vi "P2P High-Speed Stream to Disk.vi"() -> ()   [LabVIEW 2023]
doc: "Shows best-practices for streaming high-speed data to disk from a 791x coprocessor module."
uses:
  <vilib>/userDefined/Silver/nirio_resource_slv.ctl
  SubVIs/UI_indicators.ctl
  <instrlib>/_niInstr/Streaming/v1/Common/Stream State.ctl
  <vilib>/userDefined/niP2PState.ctl
  <vilib>/FPGAPlugInAG/PXIe-7915/niLvFpga_Open_PXIe-7915.vi
  <vilib>/rvi/interface/common/dynamic/niFpgaDynamicAddResources.vi
  <vilib>/FPGAPlugInAG/Dynamic/niLvFpga_P2PGetEndpoint_Dynamic.vi
  <vilib>/Utility/error.llb/Error Cluster From Error Code.vi
  <vilib>/rvi/errors/niLvFpgaAdjustHostInterfaceError.vi
  <vilib>/FPGAPlugInAG/Dynamic/niLvFpga_Close_Dynamic.vi
  <vilib>/rvi/interface/nirviOpenFPGA/nirviOpenFPGA.xnode
  FPGA Bitfiles/PXIe-791X_Getting_Started.lvbitx
  <vilib>/rvi/interface/nirviMethod/nirviMethod.xnode
  <vilib>/rvi/interface/nirviReadWriteControl/nirviReadWriteControl.xnode
  <vilib>/rvi/interface/nirviCloseFPGA/nirviCloseFPGA.xnode
  <instrlib>/_niInstr/Streaming/v1/Host/niInstr Streaming v1 Host.lvlib
  <vilib>/rvi/errors/niLvFpgaMergeErrorWithErrorCode.vi
  <instrlib>/_niInstr/Streaming/v1/Common/niInstr Streaming v1 Common.lvlib
  <instrlib>/FlexRIO/API/Host/v1/NI FlexRIO API v1.lvlib
  <resource>/objmgr/niflexrioapi.rc
  <resource>/objmgr/PeerToPeerStream.rc
  NiFpgaLv.dll
  <vilib>/rvi/interface/Simulation/niFpgaSimulationCallBeginRW.vi
  <vilib>/FPGAPlugInAG/Dynamic/niLvFpga_AcquireReadRegionFifo_Dynamic.vi
  <vilib>/FPGAPlugInAG/Dynamic/niLvFpga_StopFifo_Dynamic.vi
panel:
  out "P2P State":T1
  in  "P2P Data Source":T2="RIO1"
  out "FPGA Temperature (degC)":dbl(slide) scale=0.0..95.0
  out "Total Power Consumed (W)":dbl(slide) scale=0.0..38.25
  out "Stream Status":T3
  in  "Max File Size (GB)":dbl=2.0 format="%#_g GB"
  out "Actual Host Buffer Depth (Samples)":u32=4194304 format="%.0f S"
  in  "File Write Block Size (Samples per Read)":u32=262144 format="%.0f S"
  in  "Host Buffer Depth (# of File Write Blocks)":u32=16 format="%.0f Blocks"
  in  "TDMS File Path":path=path "C:/temp.tdms"
  in  "Total Blocks to Record (# of File Write Blocks)":u64=256 format="%.0p"
  in  "791x Coprocessor FPGA":T2="RIO0"
  # "Configuration"
  # "Power & Temperature"
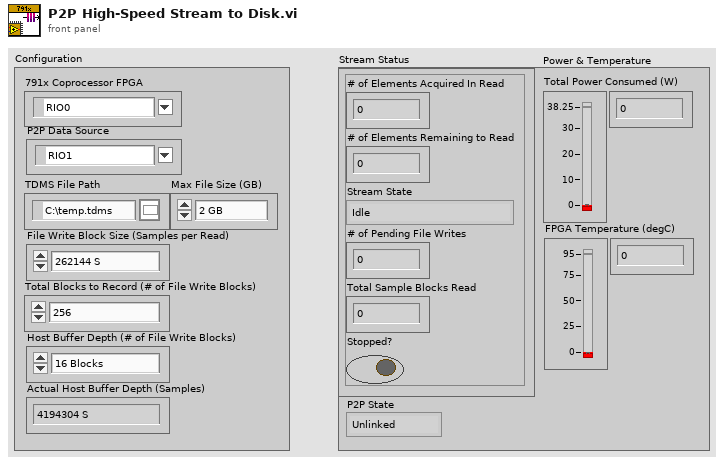
[diagram p1: front panel]
types:
  T1 = typedef "niP2PState.ctl" = enum32{"Unlinked", "Disabled", "Enabled", "Flushing"}
  T2 = typedef "nirio_resource_slv.ctl" = tag
  T3 = typedef "UI_indicators.ctl" = cluster{"# of Elements Acquired In Read":u32, "# of Elements Remaining to Read":u32, "Stream State":T4, "# of Pending File Writes":u32, "Total Sample Blocks Read":i32, "Stopped?":bool}
  T4 = typedef "niInstr Streaming v1 Common.lvlib/Stream State.ctl" = enum8{"Idle", "Finite Transfer", "Continuous", "Done", "Error", "Not Ready", "Cancel"}
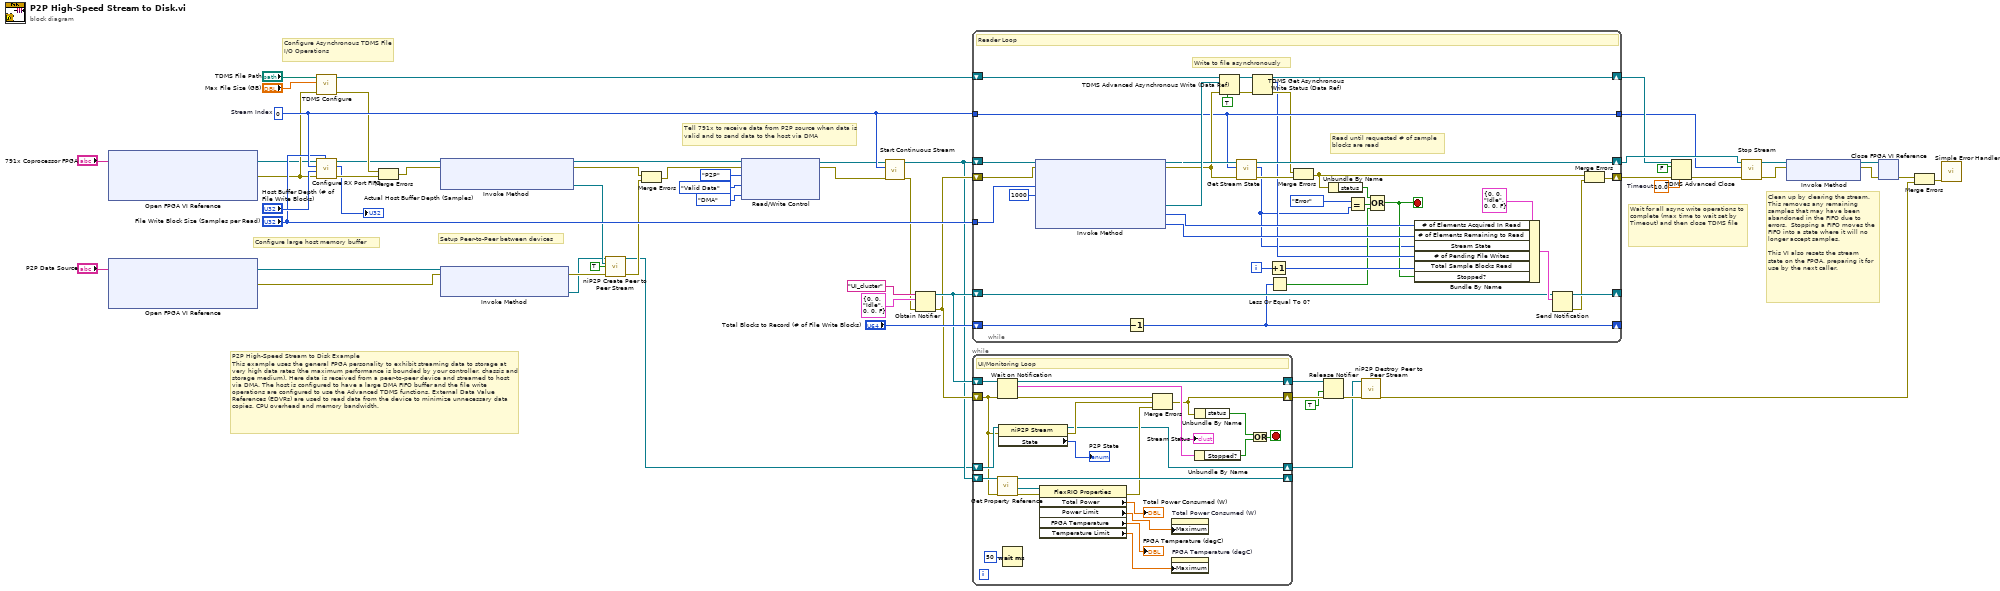
[diagram p0: block diagram]
diagram:
  w39 = 10.0  # Timeout
  w49 = 0  # Stream Index
  # "P2P High-Speed Stream to Disk Example\nThis example uses the general FPGA personality to exhibit streaming data to storage at very high data rates (the maximum performance is bounded by your controller, chassis and storage medium). Here data is received from a peer-to-peer device and streamed to host via DMA. The host is configured to have a large DMA FIFO buffer and the file write operations are configured to use the Advanced TDMS functions. External Data Value References (EDVRs) are used to read data from the device to minimize unnecessary data copies, CPU overhead and memory bandwidth."
  # "Tell 791x to receive data from P2P source when data is valid and to send data to the host via DMA"
  # "Setup Peer-to-Peer between devices"
  # "Configure large host memory buffer"
  # "Configure Asynchronous TDMS File I/O Operations"
  # "Wait for all async write operations to complete (max time to wait set by Timeout) and then close TDMS file"
  # "Clean up by clearing the stream.  This removes any remaining samples that may have been abandoned in the FIFO due to errors.  Stopping a FIFO moves the FIFO into a state where it will no longer accept samples.\n\nThis VI also resets the stream state on the FPGA, preparing it for use by the next caller."
  n1 = xnode "Open FPGA VI Reference"("resource name"="791x Coprocessor FPGA") -> ("FPGA VI Reference Out"=w22:refnum<k20>, "error out"=w25:errorcluster)  [unwired: 1 in]
  n2 = xnode "Open FPGA VI Reference"("resource name"="P2P Data Source") -> ("FPGA VI Reference Out"=w19:refnum<k20>, "error out"=w18:errorcluster)  [unwired: 1 in]
  n3 = call "TDMS Configure.vi"("error in (no error)"=w25, "Max File Size (GB)"="Max File Size (GB)", "TDMS File Path"="TDMS File Path") -> ("error out"=w47:errorcluster, "Refnum out"=w46:refnum<k34>)  [unwired: 7 in]
  n4 = call "Configure RX Port FIFO.vi"("Read Block Size (Samples per Read)"="File Write Block Size (Samples per Read)", "error in (no error)"=w25, "Host Buffer Depth (# of Read Blocks)"="Host Buffer Depth (# of File Write Blocks)", "RX Stream Index"=w49, "Refnum in"=w22) -> ("error out"=w55:errorcluster, "Actual Depth"=→"Actual Host Buffer Depth (Samples)":u32, "Refnum out"=w21:refnum<k20>)  [unwired: 4 in]
  n5 = Merge Errors(w47, w55) -> (w20:errorcluster)
  n6 = xnode "Invoke Method"("FPGA VI Reference In"=w21, "error in"=w20) -> ("FPGA VI Reference Out"=w9:refnum<k20>, "error out"=w13:errorcluster, "Reader"=w16:refnum<k20>)
  n7 = xnode "Invoke Method"("FPGA VI Reference In"=w19, "error in"=w18) -> ("error out"=w17:errorcluster, "Writer"=w15:refnum<k20>)  [unwired: 1 out]
  n8 = call <vilib>:"niP2P Create Peer to Peer Stream.vi"("writer"=w15, "reader"=w16, "enable stream (T)"=TRUE, "error in (no error)"=w17) -> ("stream session"=w4:refnum<k20>, "error out"=w12:errorcluster)  [unwired: 10 in]
  n9 = Merge Errors(w13, w12) -> (w11:errorcluster)
  n10 = xnode "Read/Write Control"("FPGA VI Reference In"=w9, "error in"=w11, "Data Source"=enum16{"DMA", "P2P"}."P2P", "Data Source Trigger"=enum16{"Valid Data", "Software"}."Valid Data", "Data Sink"=enum16{"DMA", "P2P"}."DMA") -> ("FPGA VI Reference Out"=w8:refnum<k20>, "error out"=w10:errorcluster)
  n11 = call <instrlib>:"Start Continuous Stream.vi"("error in (no error)"=w10, "stream index"=w49, "refnum in"=w8) -> ("error out"=w29:errorcluster, "refnum out"=w23:refnum<k20>)  [unwired: 7 in]
  n12 = Obtain Notifier(name (unnamed)="UI_cluster", notification data type=T3 {"# of Elements Acquired In Read"=0, "# of Elements Remaining to Read"=0, "Stream State"=enum."Idle", "# of Pending File Writes"=0, "Total Sample Blocks Read"=0, "Stopped?"=FALSE}, error in (no error)=w29) -> (notifier out=w33:refnum<notifier>, error out=w28:errorcluster)  [unwired: 1 in, 1 out]
  n13 = while {
    tunnel: w49 -> [w79]
    shift-right: [w81] -> w44
    shift-left: w23 -> [w90]
    shift-right: [w62] -> w27
    shift-left: w28 -> [w91]
    tunnel: "File Write Block Size (Samples per Read)" -> [w92]
    shift-right: [w84] -> w41
    shift-left: w46 -> [w89]
    tunnel: [w79] -> w37
    shift-right: [w72] -> _
    shift-left: w33 -> [w71]
    shift-right: [w69] -> _
    shift-left: "Total Blocks to Record (# of File Write Blocks)" -> [w70]
    i -> [w67]
    stop <- w65 stop-if-true
    # "Read until requested # of sample\nblocks are read"
    # "Write to file asynchronously"
    # "Reader Loop"
    n14 = xnode "Invoke Method"("FPGA VI Reference In"=w90, "error in"=w91, "Number of Elements"=w92, "Timeout (ms)"=1000 ("Read Timeout (ms)")) -> ("FPGA VI Reference Out"=w82:refnum<k20>, "error out"=w80:errorcluster, "Read Region Reference"=w88:refnum<data-value>, "Elements In Region"=w75:u32, "Elements Remaining"=w74:u32)
    n15 = Decrement(x=w70) -> (x-1=w69:u64)
    n16 = TDMS Advanced Asynchronous Write (Data Ref)(6:TRUE ("auto delete reference? (T)"), 8:w80, 10:w88, 11:w89) -> (0:w85:errorcluster, 3:w86:refnum<k34>)
    n17 = call <instrlib>:"Get Stream State.vi"("error in (no error)"=w80, "stream index"=w79, "refnum in"=w82) -> ("error out"=w83:errorcluster, "stream state"=w58:T4, "refnum out"=w81:refnum<k20>)  [unwired: 6 in]
    n18 = TDMS Get Asynchronous Write Status (Data Ref)(8:w85, 11:w86) -> (0:w78:errorcluster, 2:w73:u32, 3:w84:refnum<k34>)
    n19 = Increment(x=w67) -> (x+1=w66:i32)
    n20 = Less Or Equal To 0?(x=w69) -> (x <= 0?=w61:bool)
    n21 = Merge Errors(w78, w83) -> (w64:errorcluster)
    n22 = Unbundle By Name(w64) -> ("status"=w77:bool)
    n23 = Equal?(x=Stream_State."Error" ("stream state"), y=w58) -> (x = y?=w60:bool)
    n24 = Compound Arithmetic op=OR(w77, w60, w61) -> (w65:bool)
    n25 = Bundle By Name(cluster=T3 {"# of Elements Acquired In Read"=0, "# of Elements Remaining to Read"=0, "Stream State"=enum."Idle", "# of Pending File Writes"=0, "Total Sample Blocks Read"=0, "Stopped?"=FALSE}, "# of Elements Acquired In Read"=w75, "# of Elements Remaining to Read"=w74, "Stream State"=w58, "# of Pending File Writes"=w73, "Total Sample Blocks Read"=w66, "Stopped?"=w65) -> (w76:T3)
    n26 = Send Notification(notification=w76, notifier=w71) -> (notifier out=w72:refnum<notifier>, error out=w63:errorcluster)  [unwired: 1 in]
    n27 = Merge Errors(w64, w63) -> (w62:errorcluster)
  }
  n28 = while {
    shift-right: [w100] -> w32
    shift-left: w28 -> [w98]
    shift-right: [w115] -> w31
    shift-left: w33 -> [w116]
    shift-right: [w105] -> _
    shift-left: w23 -> [w108]
    shift-right: [w95] -> w2
    shift-left: w4 -> [w99]
    stop <- w109 stop-if-true
    # "UI/Monitoring Loop"
    n29 = Wait on Notification(notifier=w116, error in (no error)=w98) -> (notifier out=w115:refnum<notifier>, notification=w113:T3, error out=w112:errorcluster)  [unwired: 2 in, 1 out]
    "Stream Status" <- w113
    n30 = call <instrlib>:"Get Property Reference.vi"("fpga interface in"=w108, "error in"=w98) -> ("fpga interface out"=w105:refnum<k20>, "property reference"=w107:refnum<k20>, "error out"=w106:errorcluster)  [unwired: 11 in]
    n31 = property class="niP2P Stream"(reference=w99, error in=w98) -> (reference out=w95:refnum<k20>, error out=w96:errorcluster, "State"=→"P2P State":T1)
    n32 = Wait (ms)(milliseconds to wait=u32 50) -> ()  [unwired: 1 out]
    n33 = property class="FlexRIO Properties"(reference=w107, error in=w106) -> (error out=w97:errorcluster, "Total Power"=→"Total Power Consumed (W)":dbl, "Power Limit"=w103:dbl, "FPGA Temperature"=→"FPGA Temperature (degC)":dbl, "Temperature Limit"=w101:dbl)  [unwired: 1 out]
    n34 = Merge Errors(w112, w96, w97) -> (w100:errorcluster)
    n35 = property on="Total Power Consumed (W)" class="Slide (strict)"("Maximum"=w103) -> ()  [unwired: 2 in, 2 out]
    n36 = property on="FPGA Temperature (degC)" class="Slide (strict)"("Maximum"=w101) -> ()  [unwired: 2 in, 2 out]
    n37 = Unbundle By Name(w113) -> ("Stopped?"=w110:bool)
    n38 = Unbundle By Name(w100) -> ("status"=w111:bool)
    n39 = Or(x=w111, y=w110) -> (x .or. y?=w109:bool)
  }
  n40 = Release Notifier(notifier=w31, force destroy? (F)=TRUE, error in (no error)=w32) -> (error out=w3:errorcluster)  [unwired: 2 out]
  n41 = call <vilib>:"niP2P Destroy Peer to Peer Stream.vi"("stream session"=w2, "error in (no error)"=w3) -> ("error out"=w1:errorcluster)  [unwired: 13 in]
  n42 = TDMS Advanced Close(6:w39, 8:w27, 10:FALSE ("truncate file? (F)"), 11:w41) -> (0:w26:errorcluster)  [unwired: 1 out]
  n43 = call <instrlib>:"Stop Stream.vi"("error in (no error)"=w26, "stream index"=w37, "refnum in"=w44) -> ("error out"=w42:errorcluster, "refnum out"=w43:refnum<k20>)  [unwired: 5 in, 2 out]
  n44 = xnode "Invoke Method"("FPGA VI Reference In"=w43, "error in"=w42) -> ("FPGA VI Reference Out"=w53:refnum<k20>, "error out"=w54:errorcluster)
  n45 = xnode "Close FPGA VI Reference"("FPGA VI Reference In"=w53, "error in"=w54) -> ("error out"=w57:errorcluster)
  n46 = Merge Errors(w57, w1) -> (w38:errorcluster)
  n47 = call <vilib>:"Simple Error Handler.vi"("error in (no error)"=w38) -> ()  [unwired: 4 in, 5 out]
